vi "GraphClear.vi"() -> ()   [LabVIEW 2021]
panel:
  out "Waveform Graph":dynamicdata(graph)
  in  "stop":bool
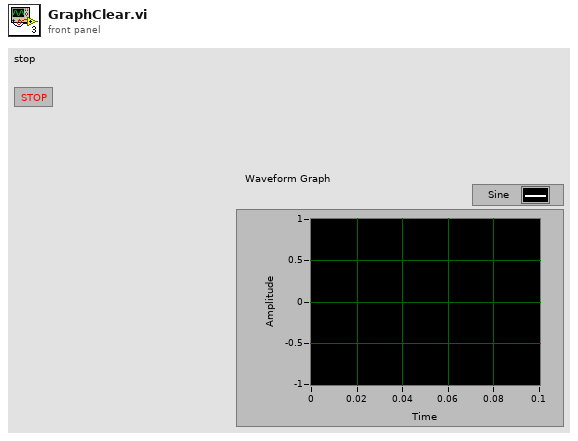
[diagram p1: front panel]
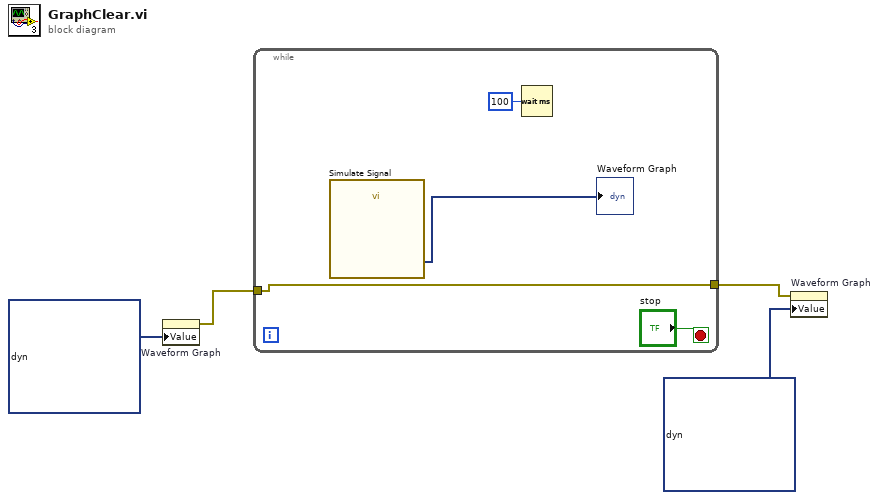
[diagram p0: block diagram]
diagram:
  n1 = property on="Waveform Graph" class="WFGraph (strict)"("Value"=dynamicdata [] ("Waveform Graph")) -> (error out=w2:errorcluster)  [unwired: 2 in, 1 out]
  n2 = while {
    tunnel: [w6] -> w3
    tunnel: w2 -> [w6]
    stop <- "stop" stop-if-true
    n3 = call "Simulate Signal"() -> ("Sine"=→"Waveform Graph":dynamicdata)  [unwired: 14 in, 1 out]
    n4 = Wait (ms)(milliseconds to wait=u32 100) -> ()  [unwired: 1 out]
  }
  n5 = property on="Waveform Graph" class="WFGraph (strict)"(error in=w3, "Value"=dynamicdata [] ("Waveform Graph")) -> ()  [unwired: 1 in, 2 out]
